vi "Brake.vi"(4 "Brake?":bool, 5 "Wheel diameter (in)":dbl, 6 "error in (no error)":errorcluster, 7 "Right Speed":dbl, 9 "Left Speed":dbl) -> (0 "error out":errorcluster, 1 "Right Output":dbl, 3 "Left Output":dbl)   [LabVIEW 2011]
uses:
  <vilib>/addons/control/pid/pid.llb/PID (DBL).vi
  <vilib>/addons/control/pid/NI_PID_pid.lvlib
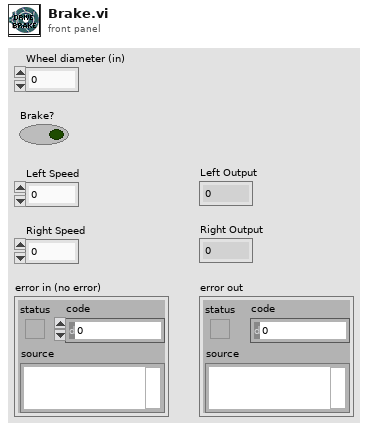
[diagram p1: front panel]
types:
  T1 = cluster{"proportional gain (Kc)":dbl, "integral time (Ti, min)":dbl, "derivative time (Td, min)":dbl}
  T2 = typedef "WPI_EncoderDevRef.ctl" = cluster{"DevStatus":errorcluster, "EncoderIndex":T3, "CounterIndex":T4, "DistancePerCount":dbl, "Decoding Type":T5}
  T3 = typedef "FPGA_EncoderIdx.ctl" = enum8{"Enc 0", "Enc 1", "Enc 2", "Enc 3", "Invalid"}
  T4 = typedef "FPGA_CounterCtrSystemIndex.ctl" = enum8{"Ctr 0", "Ctr 1", "Ctr 2", "Ctr 3", "Ctr 4", "Ctr 5", "Ctr 6", "Ctr 7", "Invalid"}
  T5 = typedef "WPI_EncoderType.ctl" = enum16{"1x", "2x", "4x"}
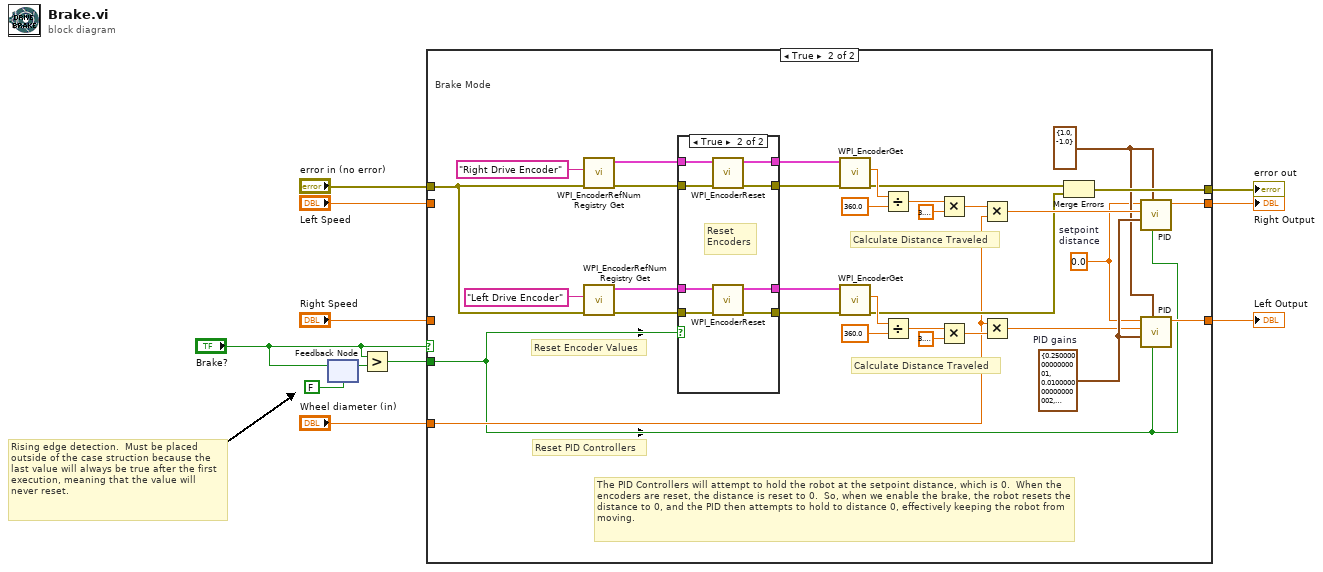
[diagram p0: block diagram]
diagram:
  # "Rising edge detection.  Must be placed outside of the case struction because the last value will always be true after the first execution, meaning that the value will never reset."
  n1 = feedback #1(FALSE) -> (w3:bool)
  n2 = feedback-in #1("Brake?") -> ()
  n3 = Greater?(x="Brake?", y=w3) -> (0:w1:bool)
  n4 = case shown="True" "Brake?" {
    tunnel: [w14 w27] -> w7
    tunnel: [w13 w26] -> w8
    tunnel: "Right Speed" -> [w14 _]
    tunnel: "Left Speed" -> [w13 _]
    tunnel: "error in (no error)" -> [w12 w23]
    tunnel: [w12 w20] -> w10
    tunnel: "Wheel diameter (in)" -> [_ w17]
    tunnel: w1 -> [_ w16]
    frame False {
      # "Normal Driving Mode"
    }
    frame True {
      w15 = 0.0  # setpoint distance
      w47 = T1 {"proportional gain (Kc)"=0.2500000000000001, "integral time (Ti, min)"=0.010000000000000002, "derivative time (Td, min)"=0.003}  # PID gains
      w18 = cluster{"output high":dbl, "output low":dbl} {"output high"=1.0, "output low"=-1.0} ("output range")
      # "The PID Controllers will attempt to hold the robot at the setpoint distance, which is 0.  When the encoders are reset, the distance is reset to 0.  So, when we enable the brake, the robot resets the distance to 0, and the PID then attempts to hold to distance 0, effectively keeping the robot from moving."
      # "Calculate Distance Traveled"
      # "Calculate Distance Traveled"
      # "Reset Encoder Values"
      # "Reset PID Controllers"
      # "Brake Mode"
      n5 = call <vilib>:"WPI_EncoderRefNum Registry Get.vi"("error in (no error)"=w23, "refnum name"="Right Drive Encoder") -> ("error out"=w29:errorcluster, "EncoderDevRef"=w33:T2)  [unwired: 8 in]
      n6 = call <vilib>:"WPI_EncoderRefNum Registry Get.vi"("error in (no error)"=w23, "refnum name"="Left Drive Encoder") -> ("error out"=w31:errorcluster, "EncoderDevRef"=w32:T2)  [unwired: 8 in]
      n7 = case shown="True" w16 {
        tunnel: [w51 w55] -> w46
        tunnel: [w49 w53] -> w39
        tunnel: w33 -> [w51 w59]
        tunnel: w32 -> [w49 w58]
        tunnel: w31 -> [w48 w57]
        tunnel: [w48 w52] -> w30
        tunnel: w29 -> [w50 w56]
        tunnel: [w50 w54] -> w28
        frame False {
        }
        frame True {
          # "Reset\nEncoders"
          n8 = call <vilib>:"WPI_EncoderReset.vi"("error in (no error)"=w56, "EncoderDevRef"=w59) -> ("error out"=w54:errorcluster, "EncoderDevRef"=w55:T2)  [unwired: 8 out]
          n9 = call <vilib>:"WPI_EncoderReset.vi"("error in (no error)"=w57, "EncoderDevRef"=w58) -> ("error out"=w52:errorcluster, "EncoderDevRef"=w53:T2)  [unwired: 8 out]
        }
      }
      n10 = call <vilib>:"WPI_EncoderGet.vi"("error in (no error)"=w28, "EncoderDevRef"=w46) -> ("error out"=w22:errorcluster, "Distance"=w41:dbl)  [unwired: 8 out]
      n11 = call <vilib>:"WPI_EncoderGet.vi"("error in (no error)"=w30, "EncoderDevRef"=w39) -> ("error out"=w21:errorcluster, "Distance"=w35:dbl)  [unwired: 8 out]
      n12 = Divide(x=w41, y=360.0) -> (x/y=w45:dbl)
      n13 = Divide(x=w35, y=360.0) -> (x/y=w38:dbl)
      n14 = Multiply(x=w45, y=3.141592653589793) -> (x*y=w44:dbl)
      n15 = Multiply(x=w38, y=3.141592653589793) -> (x*y=w19:dbl)
      n16 = Multiply(x=w44, y=w17) -> (x*y=w40:dbl)
      n17 = Multiply(x=w17, y=w19) -> (x*y=w34:dbl)
      n18 = Merge Errors(w22, w21) -> (w20:errorcluster)
      n19 = call-poly <vilib>:"PID.vi"("reinitialize? (F)"=w16, "output range"=w18, "PID gains"=w47, "process variable"=w40, "setpoint"=w15) -> ("output"=w26:dbl)  [unwired: 5 in, 1 out]
      n20 = call-poly <vilib>:"PID.vi"("reinitialize? (F)"=w16, "output range"=w18, "PID gains"=w47, "process variable"=w34, "setpoint"=w15) -> ("output"=w27:dbl)  [unwired: 5 in, 1 out]
    }
  }
  "error out" <- w10
  "Right Output" <- w8
  "Left Output" <- w7
